vi "CFG Convert String to DAQ Variant.vi"(0 "Special Instructions":string, 5 "Value String in":string="Empty", 9 "Value Variant In":variant, 11 "error in":errorcluster) -> (4 "Value Variant Out":variant, 6 "DAQmx Type":T1=enum."Terminal", 8 "Channel Signal Type":i32, 10 "Value String Out":string, 15 "error out":errorcluster)   [LabVIEW 2017]
uses:
  Type Defs/CFG DAQmx Type Enum.ctl
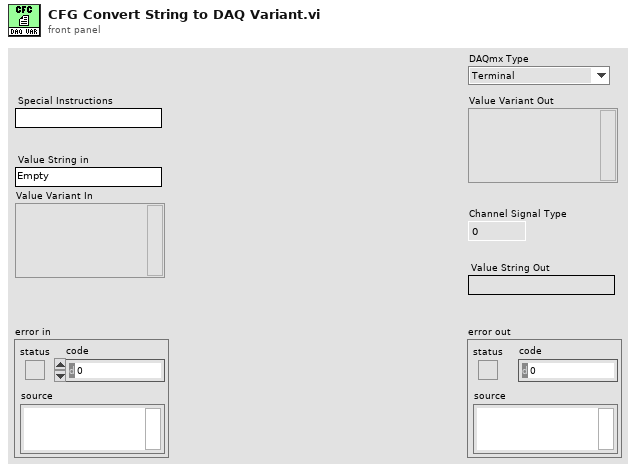
[diagram p1: front panel]
types:
  T1 = typedef "CFG DAQmx Type Enum.ctl" = enum16{"Analog Input", "Analog Output", "Digital Input", "Digital Output", "Counter Input", "Counter Output", "Terminal", ""}
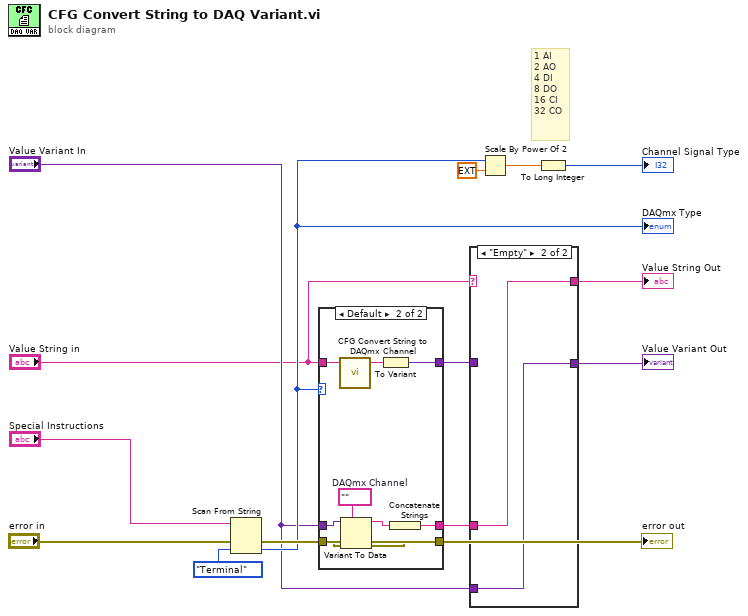
[diagram p0: block diagram]
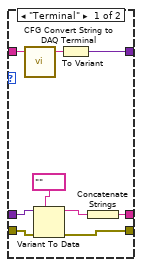
[diagram p3: hidden frame]
diagram:
  # "1 AI \n2 AO \n4 DI \n8 DO \n16 CI \n32 CO"
  n1 = Scan From String(input string="Special Instructions", error in="error in", default 1=CFG_DAQmx_Type_Enum."Terminal") -> (error out=w8:errorcluster, output 1=w7:T1)  [unwired: 2 in, 2 out]
  "error out" <- w8
  "DAQmx Type" <- w7
  n2 = case shown="Default" w7 {
    tunnel: w8 -> [w23 w29]
    tunnel: [w20 w27] -> w4
    tunnel: [w22 w28] -> _
    tunnel: "Value Variant In" -> [w19 w30]
    tunnel: "Value String in" -> [w16 w25]
    tunnel: [w15 w26] -> w1
    frame "Terminal" {
      n3 = call "CFG Convert String to DAQ Terminal.vi"("VISA String"=w16) -> ("Terminal"=w17:tag)  [unwired: 4 out]
      n4 = Variant To Data(error in=w23, type=tag "" ("Terminal"), Variant=w19) -> (data=w21:tag, error out=w22:errorcluster)
      n5 = To Variant(anything=w17) -> (Variant=w15:variant)
      n6 = Concatenate Strings(w21) -> (w20:string)
    }
    frame Default {
      w31 = tag ""  # DAQmx Channel
      n7 = call "CFG Convert String to DAQmx Channel.vi"("DAQ String"=w25) -> ("DAQmx Channel Input"=w24:tag)  [unwired: 4 out]
      n8 = Variant To Data(error in=w29, type=w31, Variant=w30) -> (data=w32:tag, error out=w28:errorcluster)
      n9 = To Variant(anything=w24) -> (Variant=w26:variant)
      n10 = Concatenate Strings(w32) -> (w27:string)
    }
  }
  n11 = case shown="\"Empty\"" "Value String in" {
    selector: "Value String in" -> [w33 _]
    tunnel: "Value Variant In" -> [_ w35]
    tunnel: [w33 w36] -> w2
    tunnel: w4 -> [_ w36]
    tunnel: [w34 w35] -> w3
    tunnel: w1 -> [w34 _]
    frame Default {
    }
    frame "Empty" {
    }
  }
  "Value Variant Out" <- w3
  "Value String Out" <- w2
  n12 = Scale By Power Of 2(n=w7, x=ext 1.0) -> (x*2^n=w11:ext)
  n13 = To Long Integer(number=w11) -> (32bit integer=→"Channel Signal Type":i32)
